vi "Hz_to_DAC.vi"(1 "Subtract":bool[](array[boolean])=[FALSE, FALSE, FALSE, FALSE, FALSE, FALSE, FALSE, FALSE], 2 "Delta":i32[](array[numeric])=[0, 0, 0, 0, 0, 0, 0, 0], 3 "Add":bool[](array[boolean])=[TRUE, TRUE, TRUE, TRUE, TRUE, TRUE, TRUE, FALSE]) -> (0 "Output counts":i32)   [LabVIEW 2014]
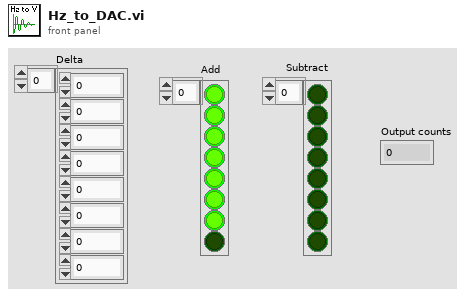
[diagram p1: front panel]
types:
  T1 = cluster{"Add[0]":bool, "Add[1]":bool, "Add[2]":bool, "Add[3]":bool, "Add[4]":bool, "Add[5]":bool, "Add[6]":bool, "Add[7]":bool}
  T2 = cluster{"Subtract[0]":bool, "Subtract[1]":bool, "Subtract[2]":bool, "Subtract[3]":bool, "Subtract[4]":bool, "Subtract[5]":bool, "Subtract[6]":bool, "Subtract[7]":bool}
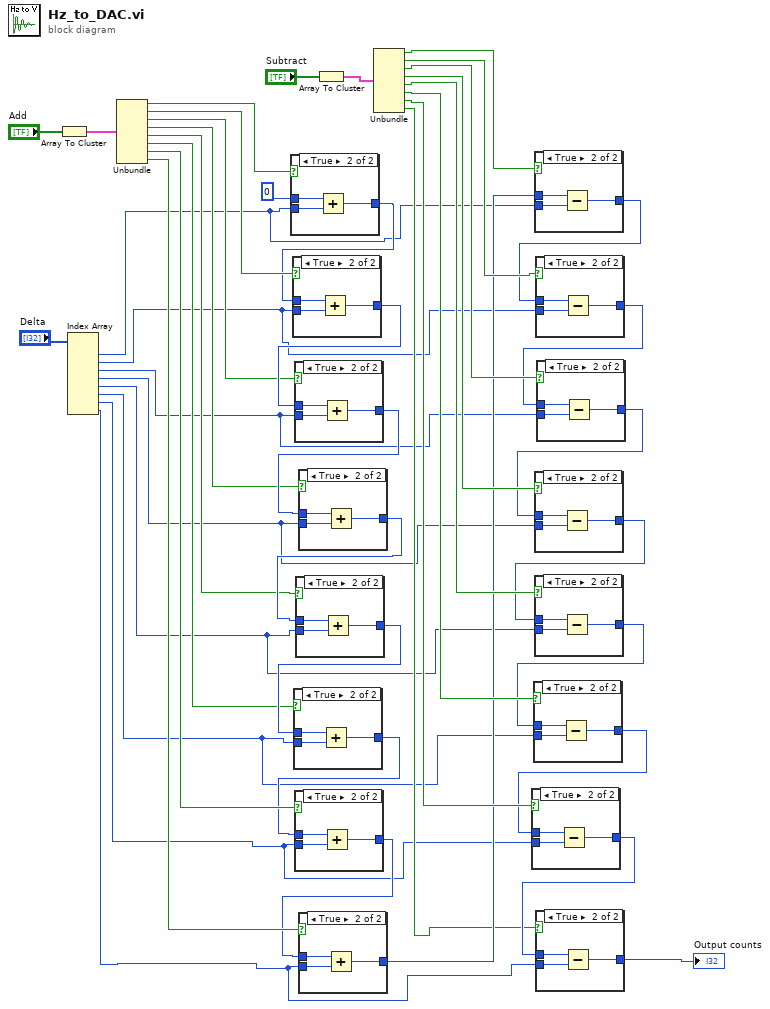
[diagram p0: block diagram]
diagram:
  n1 = Array To Cluster(array="Add") -> (cluster=w45:T1)
  n2 = Index Array(array="Delta") -> (element #1=w8:i32, element #2=w7:i32, element #3=w6:i32, element #4=w5:i32, element #5=w4:i32, element #6=w3:i32, element #7=w2:i32, element #8=w1:i32)  [unwired: 8 in]
  n3 = Unbundle(w45) -> ("Add[0]"=w44:bool, "Add[1]"=w38:bool, "Add[2]"=w37:bool, "Add[3]"=w36:bool, "Add[4]"=w35:bool, "Add[5]"=w34:bool, "Add[6]"=w33:bool, "Add[7]"=w14:bool)
  n4 = case shown="True" w44 {
    tunnel: w8 -> [_ w48]
    tunnel: [w47 w50] -> w30
    tunnel: 0 -> [w47 w49]
    frame False {
    }
    frame True {
      n5 = Add(x=w49, y=w48) -> (x+y=w50:i32)
    }
  }
  n6 = case shown="True" w38 {
    tunnel: w7 -> [_ w54]
    tunnel: [w51 w53] -> w42
    tunnel: w30 -> [w51 w52]
    frame False {
    }
    frame True {
      n7 = Add(x=w52, y=w54) -> (x+y=w53:i32)
    }
  }
  n8 = case shown="True" w37 {
    tunnel: w6 -> [_ w58]
    tunnel: [w55 w57] -> w41
    tunnel: w42 -> [w55 w56]
    frame False {
    }
    frame True {
      n9 = Add(x=w56, y=w58) -> (x+y=w57:i32)
    }
  }
  n10 = case shown="True" w36 {
    tunnel: w5 -> [_ w62]
    tunnel: [w59 w61] -> w40
    tunnel: w41 -> [w59 w60]
    frame False {
    }
    frame True {
      n11 = Add(x=w60, y=w62) -> (x+y=w61:i32)
    }
  }
  n12 = case shown="True" w35 {
    tunnel: w4 -> [_ w66]
    tunnel: [w63 w65] -> w39
    tunnel: w40 -> [w63 w64]
    frame False {
    }
    frame True {
      n13 = Add(x=w64, y=w66) -> (x+y=w65:i32)
    }
  }
  n14 = case shown="True" w34 {
    tunnel: w3 -> [_ w70]
    tunnel: [w67 w69] -> w17
    tunnel: w39 -> [w67 w68]
    frame False {
    }
    frame True {
      n15 = Add(x=w68, y=w70) -> (x+y=w69:i32)
    }
  }
  n16 = case shown="True" w33 {
    tunnel: w2 -> [_ w74]
    tunnel: [w71 w73] -> w13
    tunnel: w17 -> [w71 w72]
    frame False {
    }
    frame True {
      n17 = Add(x=w72, y=w74) -> (x+y=w73:i32)
    }
  }
  n18 = case shown="True" w14 {
    tunnel: w1 -> [_ w78]
    tunnel: [w75 w77] -> w12
    tunnel: w13 -> [w75 w76]
    frame False {
    }
    frame True {
      n19 = Add(x=w76, y=w78) -> (x+y=w77:i32)
    }
  }
  n20 = Array To Cluster(array="Subtract") -> (cluster=w31:T2)
  n21 = Unbundle(w31) -> ("Subtract[0]"=w23:bool, "Subtract[1]"=w24:bool, "Subtract[2]"=w25:bool, "Subtract[3]"=w26:bool, "Subtract[4]"=w27:bool, "Subtract[5]"=w28:bool, "Subtract[6]"=w29:bool, "Subtract[7]"=w9:bool)
  n22 = case shown="True" w23 {
    tunnel: w8 -> [_ w82]
    tunnel: [w79 w81] -> w22
    tunnel: w12 -> [w79 w80]
    frame False {
    }
    frame True {
      n23 = Subtract(x=w80, y=w82) -> (x-y=w81:i32)
    }
  }
  n24 = case shown="True" w24 {
    tunnel: w7 -> [_ w86]
    tunnel: [w83 w85] -> w21
    tunnel: w22 -> [w83 w84]
    frame False {
    }
    frame True {
      n25 = Subtract(x=w84, y=w86) -> (x-y=w85:i32)
    }
  }
  n26 = case shown="True" w25 {
    tunnel: w6 -> [_ w90]
    tunnel: [w87 w89] -> w20
    tunnel: w21 -> [w87 w88]
    frame False {
    }
    frame True {
      n27 = Subtract(x=w88, y=w90) -> (x-y=w89:i32)
    }
  }
  n28 = case shown="True" w26 {
    tunnel: w5 -> [_ w94]
    tunnel: [w91 w93] -> w19
    tunnel: w20 -> [w91 w92]
    frame False {
    }
    frame True {
      n29 = Subtract(x=w92, y=w94) -> (x-y=w93:i32)
    }
  }
  n30 = case shown="True" w27 {
    tunnel: w4 -> [_ w98]
    tunnel: [w95 w97] -> w18
    tunnel: w19 -> [w95 w96]
    frame False {
    }
    frame True {
      n31 = Subtract(x=w96, y=w98) -> (x-y=w97:i32)
    }
  }
  n32 = case shown="True" w28 {
    tunnel: w3 -> [_ w102]
    tunnel: [w99 w101] -> w16
    tunnel: w18 -> [w99 w100]
    frame False {
    }
    frame True {
      n33 = Subtract(x=w100, y=w102) -> (x-y=w101:i32)
    }
  }
  n34 = case shown="True" w29 {
    tunnel: w2 -> [_ w106]
    tunnel: [w103 w105] -> w10
    tunnel: w16 -> [w103 w104]
    frame False {
    }
    frame True {
      n35 = Subtract(x=w104, y=w106) -> (x-y=w105:i32)
    }
  }
  n36 = case shown="True" w9 {
    tunnel: w1 -> [_ w110]
    tunnel: [w107 w109] -> w11
    tunnel: w10 -> [w107 w108]
    frame False {
    }
    frame True {
      n37 = Subtract(x=w108, y=w110) -> (x-y=w109:i32)
    }
  }
  "Output counts" <- w11
